vi "test_ThreeSessThreePinTwoInstrTwoSiteReservation_CallGetConnectionFromPinForAllDcPowerPinsOneSite_ReturnsOneConnection.vi"(8 "error in":errorcluster) -> (0 "error out":errorcluster, 2 "result":string, 3 "pass":bool)   [LabVIEW 2020, in "MeasurementServerTests.lvlib"]
uses:
  MeasurementServerTests.lvlib
  Runtime/APIs/Session Management V1/Session Reservation/Connection.ctl
  Runtime/APIs/Session Management V1/Session Reservation/Session Reservation.lvclass
  Runtime/APIs/Session Management V1/Session Reservation/Connection with Session.ctl
  cd6edcbc-9d4b-497e-9505-409c6efc4fd9.vi
  78747cdb-528d-4699-bbb8-5f80a429bdfd.vi
  Runtime/Sessions/niDCPower Sessions/Session Factory/Session Factory.lvclass
  Runtime/APIs/Session Management V1/Session Reservation/Pin Type.ctl
  f4a4144c-1eaa-466c-9caf-971ca4f768c7.vi
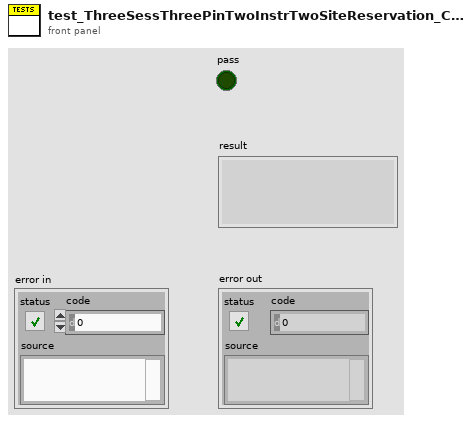
[diagram p1: front panel]
types:
  T1 = typedef "Plug-In SDK Session Management V1.lvlib/Session Reservation.lvclass/Pin Type.ctl" = enum16{"DUT and System Pins", "System Pins"}
  T2 = typedef "Plug-In SDK Session Management V1.lvlib/Session Reservation.lvclass/Connection.ctl" = cluster{"pin or relay name":string, "site":i32, "instrument type id":string, "channel":string}
  T3 = typedef "Plug-In SDK Session Management V1.lvlib/Session Reservation.lvclass/Connection with Session.ctl" = cluster{"connection":T2, "session":variant}
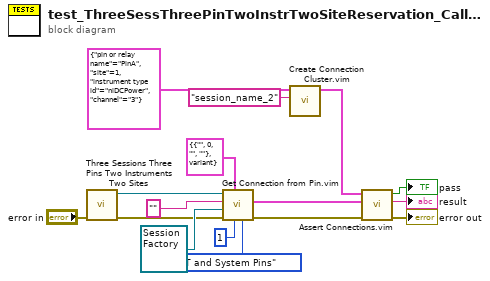
[diagram p0: block diagram]
diagram:
  n1 = call "Three Sessions Three Pins Two Instruments Two Sites.vi"("error in"="error in") -> ("error out"=w4:errorcluster, "session reservation out"=w3:refnum<class "Session Reservation.lvclass">)  [unwired: 8 in, 1 out]
  n2 = call "Get Connection from Pin.vim"("pin type"=Pin_Type."DUT and System Pins", "site"=1, "connection type"=T3 {"connection"={"pin or relay name"="", "site"=0, "instrument type id"="", "channel"=""}, "session"=variant} ("connection"), "error in"=w4, "session factory"=refnum<class "Session Factory.lvclass"> refnum ("MeasurementLink niDCPower.lvlib:Instrument.lvclass"), "pin or relay name"="", "session reservation in"=w3) -> ("error out"=w2:errorcluster, "connection"=w16:T3)  [unwired: 2 in, 1 out]
  n3 = call "Create Connection Cluster.vim"("session in"="session_name_2", "hardware independent connection in"=T2 {"pin or relay name"="PinA", "site"=1, "instrument type id"="niDCPower", "channel"="3"} ("connection")) -> ("connection out"=w13:T3)  [unwired: 9 in]
  n4 = call "Assert Connections.vim"("error in"=w2, "actual connections"=w16, "expected connections"=w13) -> ("error out"=→"error out":errorcluster, "result"=→"result":string, "pass"=→"pass":bool)  [unwired: 6 in]
